vi "findAndTargetNeuronsNew.vi"() -> ()   [LabVIEW 2017]
uses:
  opencvSegmentConvertCoordinates-multiFrames.vi
  opencvSegmentConvertCoordinates-singleFrame.vi
  opencvSelectCandidateNeurons5Planes.vi
  opencvSegment.vi
  getComputerName.vi
  globalDevices.vi
  globalUtilities.vi
panel:
  in  "piezo1":dbl
  in  "piezo2":dbl
  in  "y":dbl
  in  "Numeric":i32=10 min=1
  in  "scale":dbl[](array[numeric])=[0.8, 0.5, 0.3]
  in  "lambda":dbl[](array[numeric])=[0.0, 0.0, 0.0]
  in  "stop 2":bool
  in  "stop":bool
  out "XY":u16[][][](array[numeric])
  out "XYZ":i32[][](array[numeric])
  out "curr. piezo pos (index)":i32
  in  "piezo M-1":i32=20
  in  "frames per second":dbl=20.0
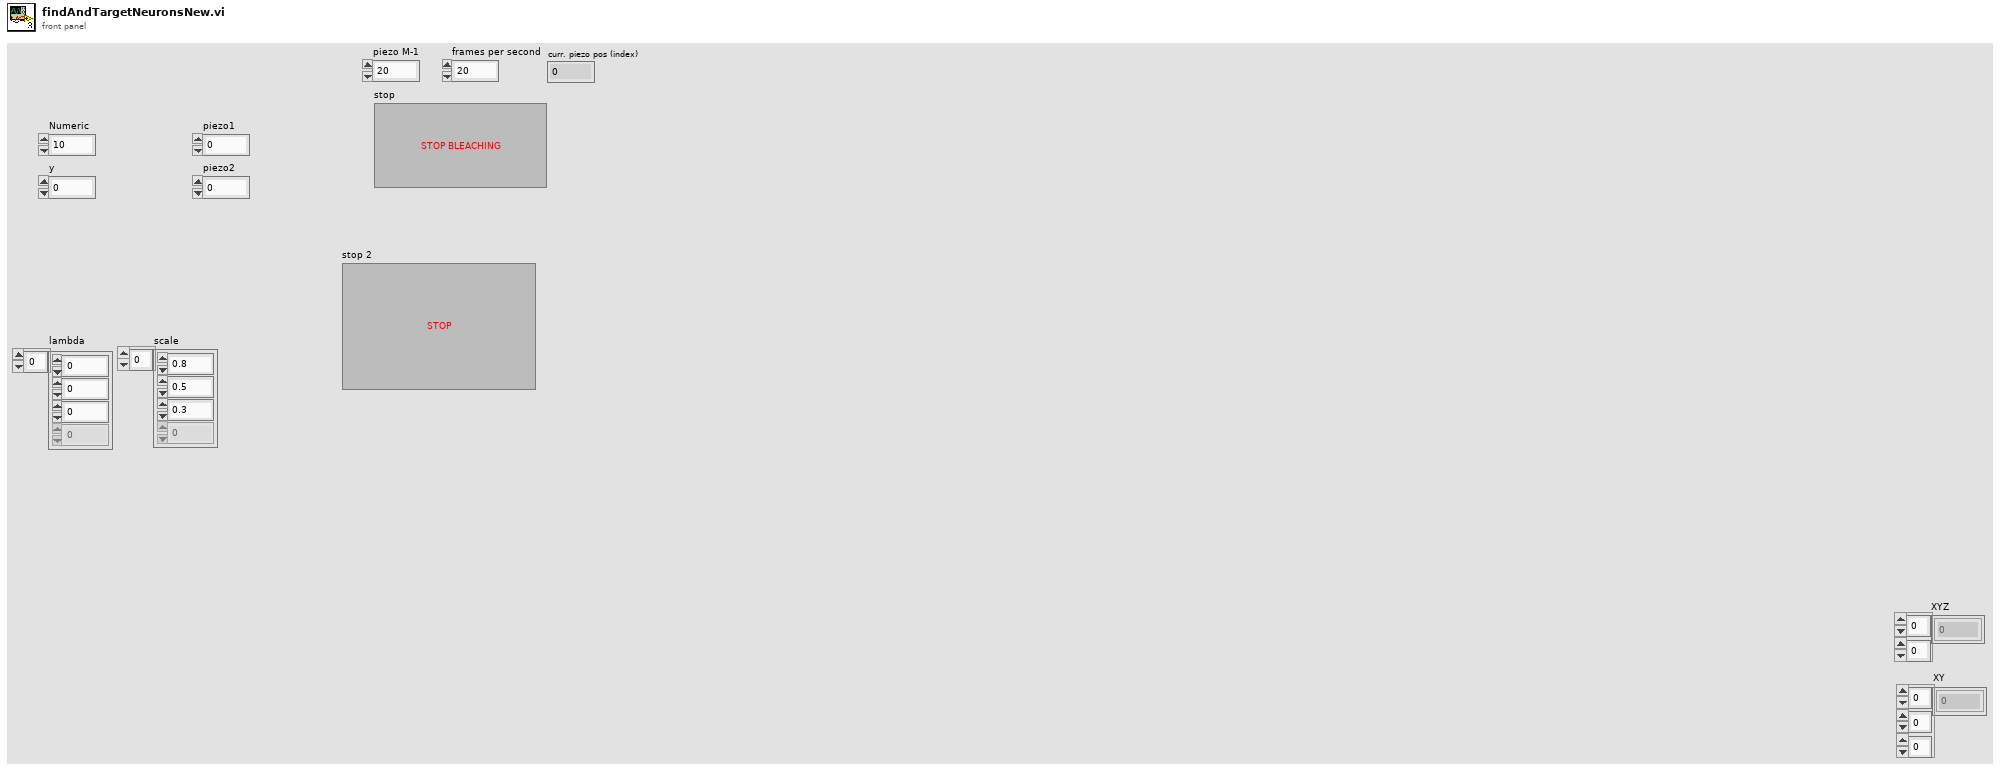
[diagram p1: front panel]
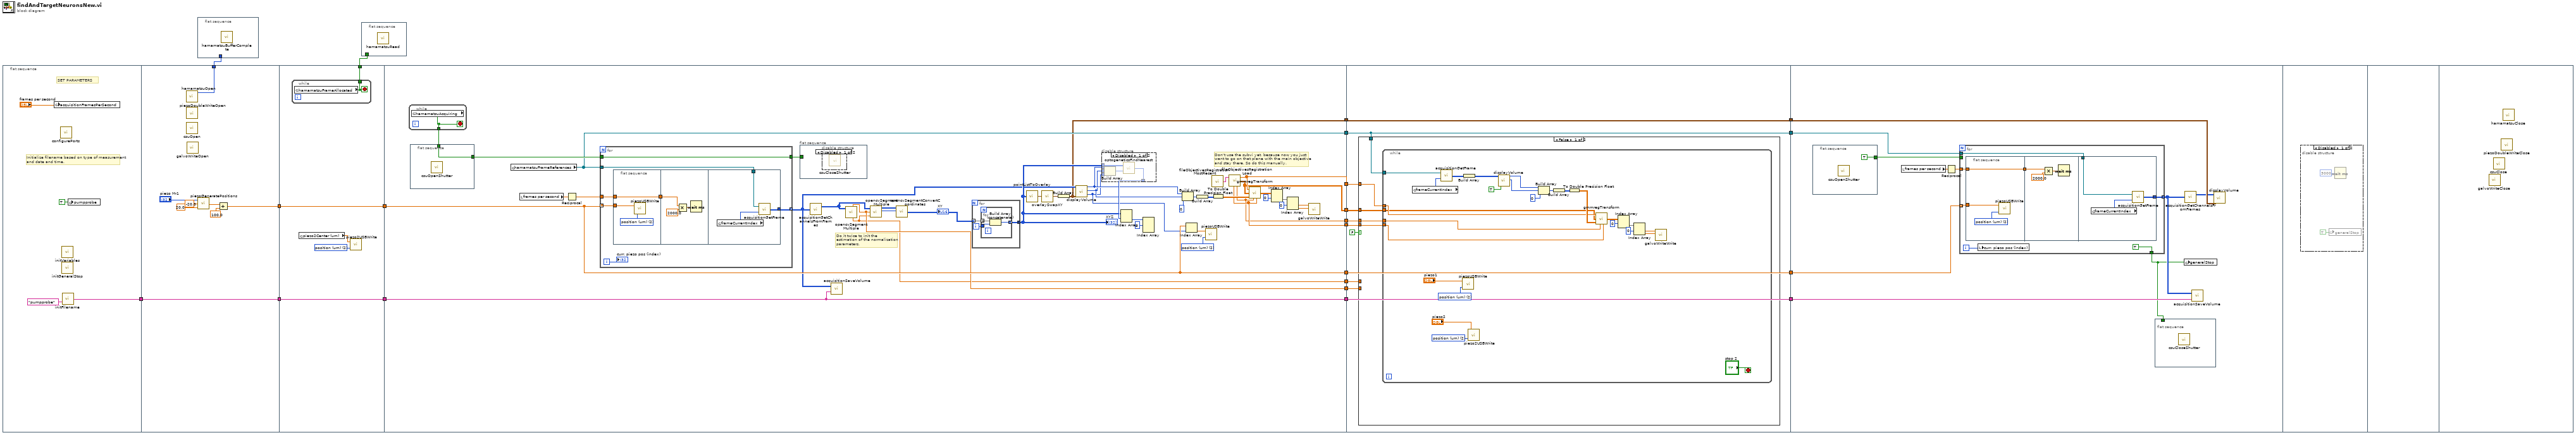
[diagram p0: block diagram]
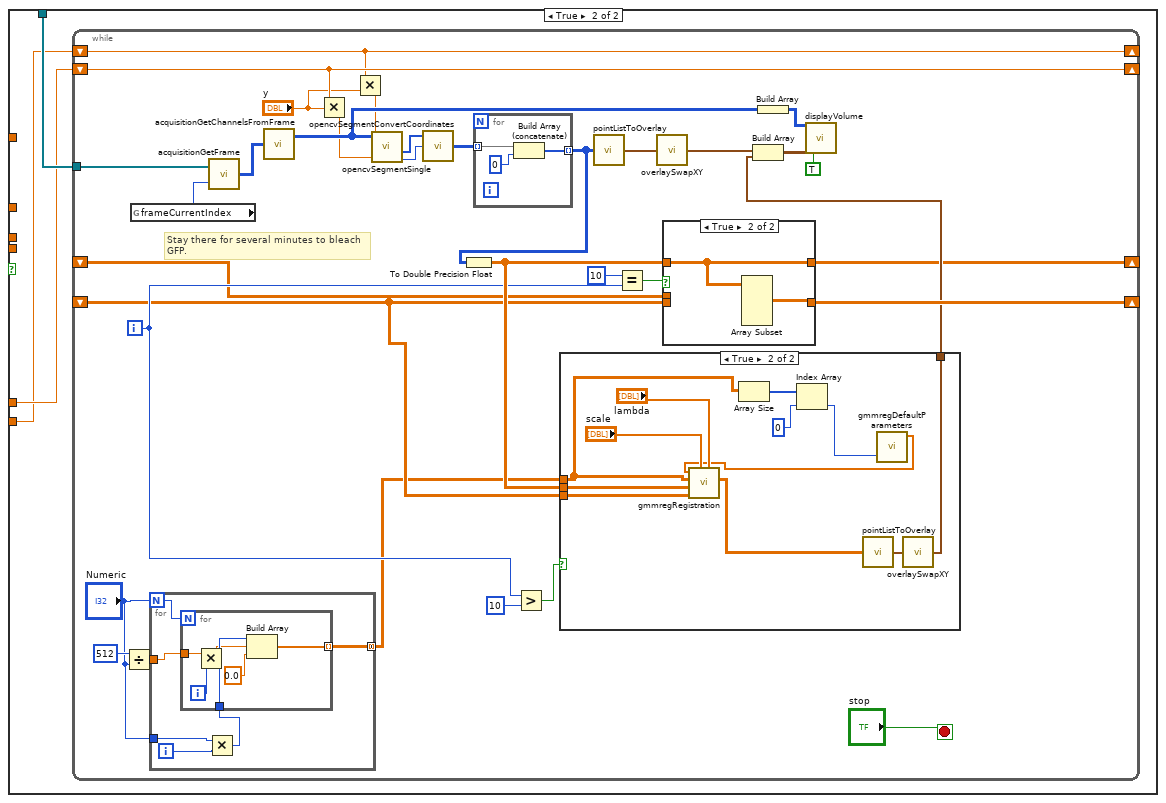
[diagram p4: hidden frame]
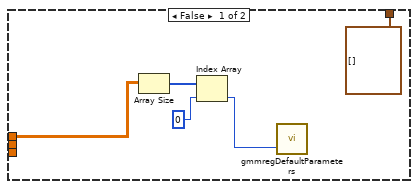
[diagram p5: hidden frame]
diagram:
  n1 = flat-sequence {
    tunnel: [w23] -> w16
    tunnel: [w28] -> w21
    tunnel: [w27] -> w19
    tunnel: [w26] -> w17
    tunnel: w16 -> [w26]
    tunnel: [w36] -> w20
    tunnel: w19 -> [w36]
    tunnel: [w35] -> w18
    tunnel: w17 -> [w35]
    tunnel: [w34] -> w7
    tunnel: w20 -> [w54]
    tunnel: w18 -> [w53]
    tunnel: [w55] -> w14
    tunnel: [w54] -> w12
    tunnel: [w53] -> w11
    tunnel: [w44] -> w9
    tunnel: [w46] -> w6
    tunnel: [w47] -> w5
    tunnel: [w43] -> w4
    tunnel: [w42] -> w3
    tunnel: [w41] -> w2
    tunnel: [w40] -> w1
    tunnel: [w120] -> w15
    tunnel: w14 -> [w120]
    tunnel: [w112] -> w13
    tunnel: w12 -> [w112]
    tunnel: w11 -> [w122]
    tunnel: [w122] -> w10
    tunnel: w9 -> [w121]
    tunnel: [w121] -> w8
    tunnel: w6 -> [w119]
    tunnel: w5 -> [w118]
    tunnel: w4 -> [w116]
    tunnel: w3 -> [w115]
    tunnel: w2 -> [w114]
    tunnel: w1 -> [w113]
    tunnel: w15 -> [w236]
    tunnel: w13 -> [w235]
    tunnel: w10 -> [w234]
    tunnel: w8 -> [w233]
    frame #0 {
      # "SET PARAMETERS"
      # "Initialize filename based on type of measurement\nand date and time."
      n2 = global write "globalUtilities.vi" "acquisitionFramesPerSecond"("frames per second") -> ()
      n3 = call "configurePorts.vi"() -> ()  [unwired: 12 in]
      n4 = call "initVariables.vi"() -> ()  [unwired: 12 in]
      n5 = call "initGeneralStop.vi"() -> ()  [unwired: 1 in]
      n6 = call "initFilename.vi"("Experiment type"="pumpprobe") -> ("folder name"=w23:string)  [unwired: 1 in]
      n7 = global write "globalUtilities.vi" "pumpprobe"(TRUE ("pumpprobe")) -> ()
    }
    frame #1 {
      n8 = call "hamamatsuOpen.vi"() -> ("Handle out"=w28:u32)  [unwired: 3 out]
      n9 = call "piezoDoubleWriteOpen.vi"() -> ()  [unwired: 2 in]
      n10 = call "csuOpen.vi"() -> ()  [unwired: 14 in, 2 out]
      n11 = call "galvoWriteOpen.vi"() -> ()  [unwired: 12 in]
      n12 = call "piezoGeneratePositions.vi"("zf"=20.0, "z0"=-20.0, "M"="piezo M-1") -> ("positions (z)"=w30:dbl[])
      n13 = Add(x=w30, y=100.0) -> (x+y=w27:dbl[])
    }
    frame #2 {
      w38 = u16 2 items=["fractional", "voltage (V)", "position (um)"] ("mode")
      n14 = while {
        tunnel: [w39] -> w34
        stop <- w39 stop-if-true
        n15 = global read "globalDevices.vi" "hamamatsuFrameAllocated"() -> (w39:bool)
      }
      n16 = global read "globalDevices.vi" "piezo2Center (um)"() -> (w37:dbl)
      n17 = call "piezo2USBWrite.vi"("mode"=w38, "position"=w37) -> ()  [unwired: 1 in]
    }
    frame #3 {
      w68 = u16 2 items=["fractional", "voltage (V)", "position (um)"] ("mode")
      # "Don't use the subvi yet, because now you just\nwant to go on that plane with the main objective\nand stay there. So do this manually."
      # "Do it twice to init the\nestimation of the normalization \nparameters."
      n18 = while {
        tunnel: [w111] -> w77
        stop <- w111 stop-if-true
        n19 = global read "globalUtilities.vi" "hamamatsuAcquiring"() -> (w111:bool)
      }
      n20 = flat-sequence {
        tunnel: w77 -> [w88]
        tunnel: [w88] -> w76
        frame #0 {
          n21 = call "csuOpenShutter.vi"() -> ()  [unwired: 16 in]
        }
      }
      n22 = global read "globalDevices.vi" "hamamatsuFrameReferences"() -> (w55:refnum<data-value>[])
      n23 = local read "frames per second"() -> (w81:dbl)
      n24 = Reciprocal(x=w81) -> (1/x=w80:dbl)
      n25 = for {
        tunnel: w55 -> [w100]
        tunnel: w54 -> [w101] mode=indexing
        tunnel: w80 -> [w99]
        tunnel: [w97] -> w48 mode=indexing
        tunnel: w76 -> [w95]
        tunnel: [w95] -> w75
        i -> [w96]
        n26 = flat-sequence {
          tunnel: w101 -> [w103]
          tunnel: w99 -> [w104]
          tunnel: [w104] -> w98
          tunnel: w98 -> [w105]
          tunnel: w100 -> [w109]
          tunnel: [w108] -> w97
          frame #0 {
            w102 = u16 2 items=["fractional", "voltage (V)", "position (um)"] ("mode")
            n27 = call "piezoUSBWrite.vi"("mode"=w102, "position"=w103) -> ()  [unwired: 1 in]
          }
          frame #1 {
            n28 = Multiply(x=w105, y=2000.0) -> (x*y=w107:dbl)
            n29 = Wait (ms)(milliseconds to wait=w107) -> ()  [unwired: 1 out]
          }
          frame #2 {
            n30 = global read "globalUtilities.vi" "frameCurrentIndex"() -> (w110:i32)
            n31 = call "acquisitionGetFrame.vi"("index"=w110, "hamamatsuFrameReferences"=w109) -> ("frameOut"=w108:u16[][])
          }
        }
        "curr. piezo pos (index)" <- w96
      }
      n32 = flat-sequence {
        tunnel: w75 -> [_]
        frame #0 {
          n33 = disable-structure shown="Disabled" {
            frame Disabled {
              n34 = call "csuCloseShutter.vi"() -> ()  [unwired: 16 in]
            }
            frame Enabled {
            }
          }
        }
      }
      n35 = call "acquisitionGetChannelsFromFrames.vi"("frameIn"=w48) -> ("Red"=w73:u16[][][])  [unwired: 1 out]
      n36 = call "acquisitionSaveVolume.vi"("folder"=w53, "volume"=w48) -> ()  [unwired: 1 in]
      n37 = call "opencvSegmentMultiple.vi"("ImgIn"=w73) -> ("maxY"=w46:dbl, "maxX"=w47:dbl)  [unwired: 2 in, 4 out]
      n38 = call "opencvSegmentMultiple.vi"("maxYInStack"=w46, "maxXInStack"=w47, "ImgIn"=w73) -> ("NeuronN[frame]"=w79:u16[], "NeuronXY[frame]"=w78:u16[][])  [unwired: 4 out]
      n39 = call-poly "opencvSegmentConvertCoordinates.vi"("NeuronN"=w79, "NeuronXY"=w78) -> ("XY"=w74:u16[][][])  [unwired: 1 in]
      "XY" <- w74
      n40 = for {
        tunnel: w74 -> [w91] mode=indexing
        tunnel: [w90] -> w71 mode=concatenating
        i -> [w89]
        n41 = for {
          tunnel: w91 -> [w94] mode=indexing
          tunnel: [w92] -> w90 mode=indexing
          tunnel: w89 -> [w93]
          n42 = Build Array (concatenate)(w94, w93) -> (w92:i32[])
        }
      }
      "XYZ" <- w71
      n43 = call "pointListToOverlay.vi"("points"=w71) -> ("overlay (XYZ)"=w49:cluster{"X":i32, "Y":i32, "Z":i32}[])
      n44 = call "overlaySwapXY.vi"("overlay in"=w49) -> ("overlay out"=w45:cluster{"X":i32, "Y":i32, "Z":i32}[])
      n45 = Build Array(w45) -> (w44:cluster{"X":i32, "Y":i32, "Z":i32}[][])
      n46 = call "displayVolume.vi"("frames"=w48, "overlay (z:-1 all planes)"=w44) -> ("X0out"=w52:i32, "Y0out"=w51:i32, "zout (plane index)"=w50:i32)  [unwired: 12 in, 3 out]
      n47 = disable-structure shown="Disabled" {
        disable-tunnel: w52 -> [w87 _]
        disable-tunnel: w51 -> [w86 _]
        disable-tunnel: w50 -> [w85 _]
        disable-tunnel: [w83 _] -> w72
        disable-tunnel: w71 -> [w82 _]
        frame Disabled {
          n48 = Build Array(w87, w86, w85) -> (w84:i32[])
          n49 = call "optogeneticsFindNearest.vi"("point"=w84, "points"=w82) -> ("min index(es)"=w83:i32)
        }
        frame Enabled {
        }
      }
      n50 = Index Array(array=w71, index (row)=w72) -> (element=w70:i32[])  [unwired: 1 in]
      n51 = Index Array(array=w70, index #1=0 ("index")) -> ()  [unwired: 2 in, 3 out]
      n52 = Build Array(w52, w51, 0 ("element")) -> (w64:i32[])
      n53 = Index Array(array=w54, index=w50) -> (element=w69:dbl)
      n54 = Build Array(w64) -> (w63:i32[][])
      n55 = call "piezoUSBWrite.vi"("mode"=w68, "position"=w69) -> ()  [unwired: 1 in]
      n56 = call "fileObjectivesRegistrationMostRecent.vi"() -> ("f"=w67:string)  [unwired: 1 in]
      n57 = To Double Precision Float(number=w63) -> (double precision float=w62:dbl[][])
      n58 = call "fileObjectivesRegistrationLoad.vi"("objectiveRegistrationFilePath"=w67) -> ("denormParam"=w41:dbl[], "param"=w43:dbl[], "imaging (model)"=w42:dbl[][], "normParam"=w40:dbl[])  [unwired: 3 in, 2 out]
      n59 = call "gmmregTransform.vi"("param0"=w43, "ctrlPts"=w42, "pts"=w62, "normParams"=w40, "denormParams"=w41) -> ("out"=w61:dbl[][])  [unwired: 4 in]
      n60 = Index Array(array=w61, index (row)=0) -> (element=w59:dbl[])  [unwired: 1 in]
      n61 = Index Array(array=w59, index #1=0 ("index")) -> (element #1=w57:dbl, element #2=w56:dbl)  [unwired: 1 in]
      n62 = call "galvoWriteWrite.vi"("X"=w57, "Y"=w56) -> ()  [unwired: 4 in]
    }
    frame #4 {
      n63 = case shown="False" FALSE {
        tunnel: w120 -> [w127 w156]
        tunnel: w119 -> [_ w155]
        tunnel: w118 -> [_ w154]
        tunnel: w116 -> [w126 _]
        tunnel: w115 -> [w125 _]
        tunnel: w114 -> [w124 _]
        tunnel: w113 -> [w123 _]
        frame False {
          n64 = while {
            tunnel: w127 -> [w151]
            tunnel: w126 -> [w138]
            tunnel: w125 -> [w137]
            tunnel: w124 -> [w135]
            tunnel: w123 -> [w136]
            stop <- "stop 2" stop-if-true
            w129 = u16 2 items=["fractional", "voltage (V)", "position (um)"] ("mode")
            w131 = u16 2 items=["fractional", "voltage (V)", "position (um)"] ("mode")
            n65 = global read "globalUtilities.vi" "frameCurrentIndex"() -> (w152:i32)
            n66 = call "acquisitionGetFrame.vi"("index"=w152, "hamamatsuFrameReferences"=w151) -> ("frameOut"=w150:u16[][])
            n67 = call "piezoUSBWrite.vi"("mode"=w131, "position"="piezo1") -> ()  [unwired: 1 in]
            n68 = Build Array(w150) -> (w149:u16[][][])
            n69 = call "piezo2USBWrite.vi"("mode"=w129, "position"="piezo2") -> ()  [unwired: 1 in]
            n70 = call "displayVolume.vi"("frames"=w149, "stop immediately"=TRUE) -> ("X0out"=w134:i32, "Y0out"=w133:i32)  [unwired: 12 in, 4 out]
            n71 = Build Array(w134, w133, 0 ("element")) -> (w140:i32[])
            n72 = Build Array(w140) -> (w141:i32[][])
            n73 = To Double Precision Float(number=w141) -> (double precision float=w142:dbl[][])
            n74 = call "gmmregTransform.vi"("param0"=w138, "ctrlPts"=w137, "pts"=w142, "normParams"=w136, "denormParams"=w135) -> ("out"=w143:dbl[][])  [unwired: 4 in]
            n75 = Index Array(array=w143, index (row)=0) -> (element=w145:dbl[])  [unwired: 1 in]
            n76 = Index Array(array=w145, index #1=0 ("index")) -> (element #1=w147:dbl, element #2=w148:dbl)  [unwired: 1 in]
            n77 = call "galvoWriteWrite.vi"("X"=w147, "Y"=w148) -> ()  [unwired: 4 in]
          }
        }
        frame True {
          n78 = while {
            tunnel: w156 -> [w188]
            shift-right: [w160] -> _
            shift-left: w154 -> [w160]
            shift-right: [w161] -> _
            shift-left: w155 -> [w161]
            shift-right: [w172] -> _
            shift-left: _ -> [w167]
            shift-right: [w177] -> _
            shift-left: _ -> [w166]
            i -> [w170]
            stop <- "stop" stop-if-true
            # "Stay there for several minutes to bleach\nGFP."
            n79 = Divide(x=512, y="Numeric") -> (x/y=w164:dbl)
            n80 = global read "globalUtilities.vi" "frameCurrentIndex"() -> (w189:i32)
            n81 = for {
              N: "Numeric" -> [w196]
              tunnel: w164 -> [w195]
              tunnel: "Numeric" -> [w193]
              tunnel: [w191] -> w162 mode=concatenating
              i -> [w194]
              n82 = Multiply(x=w193, y=w194) -> (x*y=w192:i32)
              n83 = for {
                N: w196 -> [_]
                tunnel: w192 -> [w200]
                tunnel: w195 -> [w198]
                tunnel: [w197] -> w191 mode=indexing
                i -> [w201]
                n84 = Multiply(x=w198, y=w201) -> (x*y=w199:dbl)
                n85 = Build Array(w200, w199, 0.0 ("element")) -> (w197:dbl[])
              }
            }
            n86 = call "acquisitionGetFrame.vi"("index"=w189, "hamamatsuFrameReferences"=w188) -> ("frameOut"=w187:u16[][])
            n87 = call "acquisitionGetChannelsFromFrame.vi"("frameIn"=w187) -> ("Red"=w184:u16[][])  [unwired: 1 out]
            n88 = Multiply(x=w161, y="y") -> (x*y=w158:dbl)
            n89 = Multiply(x=w160, y="y") -> (x*y=w159:dbl)
            n90 = call "opencvSegmentSingle.vi"("maxYInStack"=w158, "maxXInStack"=w159, "ImgIn"=w184) -> ("NeuronN[last frame]"=w181:u16, "NeuronXY[last frame]"=w182:u16[])  [unwired: 2 in, 2 out]
            n91 = call-poly "opencvSegmentConvertCoordinates.vi"("NeuronN"=w181, "NeuronXY"=w182) -> ("XY"=w180:u16[][])  [unwired: 1 in]
            n92 = for {
              tunnel: w180 -> [w226] mode=indexing
              tunnel: [w224] -> w173 mode=indexing
              n93 = Build Array (concatenate)(w226, 0) -> (w224:i32[])
            }
            n94 = To Double Precision Float(number=w173) -> (double precision float=w178:dbl[][])
            n95 = Greater?(x=w170, y=10) -> (0:w168:bool)
            n96 = case shown="True" w168 {
              tunnel: w178 -> [_ w218]
              tunnel: w162 -> [w203 w209]
              tunnel: w166 -> [_ w217]
              tunnel: [cluster{"X":i32, "Y":i32, "Z":i32}[] [] ("overlay out") w215] -> w175
              frame False {
                n97 = Array Size(array=w203) -> (size(s)=w206:i32[])
                n98 = Index Array(array=w206, index=0 ("index (row)")) -> (element=w204:i32)
                n99 = call "gmmregDefaultParameters.vi"("nctrlPts"=w204) -> ()  [unwired: 1 in, 4 out]
              }
              frame True {
                n100 = Array Size(array=w209) -> (size(s)=w212:i32[])
                n101 = Index Array(array=w212, index=0 ("index (row)")) -> (element=w210:i32)
                n102 = call "gmmregDefaultParameters.vi"("nctrlPts"=w210) -> ("param0"=w208:dbl[])  [unwired: 1 in, 3 out]
                n103 = call "gmmregRegistration.vi"("lambda"="lambda", "scale"="scale", "scene"=w217, "model"=w218, "ctrlPoints"=w209, "param0"=w208) -> ("out"=w214:dbl[][])  [unwired: 2 in, 3 out]
                n104 = call "pointListToOverlay.vi"("points"=w214) -> ("overlay (XYZ)"=w216:cluster{"X":i32, "Y":i32, "Z":i32}[])
                n105 = call "overlaySwapXY.vi"("overlay in"=w216) -> ("overlay out"=w215:cluster{"X":i32, "Y":i32, "Z":i32}[])
              }
            }
            n106 = call "pointListToOverlay.vi"("points"=w173) -> ("overlay (XYZ)"=w186:cluster{"X":i32, "Y":i32, "Z":i32}[])
            n107 = Equal?(x=10, y=w170) -> (x = y?=w179:bool)
            n108 = call "overlaySwapXY.vi"("overlay in"=w186) -> ("overlay out"=w176:cluster{"X":i32, "Y":i32, "Z":i32}[])
            n109 = case shown="True" w179 {
              tunnel: w178 -> [_ w223]
              tunnel: [w221 w223] -> w172
              tunnel: w167 -> [w221 _]
              tunnel: [w220 w222] -> w177
              tunnel: w166 -> [w220 _]
              frame False {
              }
              frame True {
                n110 = Array Subset(array=w223) -> (w222:dbl[][])  [unwired: 4 in]
              }
            }
            n111 = Build Array(w176, w175) -> (w174:cluster{"X":i32, "Y":i32, "Z":i32}[][])
            n112 = Build Array(w184) -> (w183:u16[][][])
            n113 = call "displayVolume.vi"("frames"=w183, "overlay (z:-1 all planes)"=w174, "stop immediately"=TRUE) -> ()  [unwired: 11 in, 6 out]
          }
        }
      }
    }
    frame #5 {
      n114 = flat-sequence {
        tunnel: [TRUE] -> w228
        frame #0 {
          n115 = call "csuOpenShutter.vi"() -> ()  [unwired: 16 in]
        }
      }
      n116 = local read "frames per second"() -> (w232:dbl)
      n117 = Reciprocal(x=w232) -> (1/x=w231:dbl)
      n118 = for {
        tunnel: w236 -> [w240]
        tunnel: w231 -> [w241]
        tunnel: w235 -> [w243] mode=indexing
        tunnel: [w239] -> w230 mode=indexing
        tunnel: [TRUE] -> w227
        tunnel: w228 -> [_]
        i -> [w238]
        n119 = flat-sequence {
          tunnel: w243 -> [w245]
          tunnel: [w244] -> w242
          tunnel: w241 -> [w244]
          tunnel: w242 -> [w249]
          tunnel: w240 -> [w251]
          tunnel: [w250] -> w239
          frame #0 {
            w246 = u16 2 items=["fractional", "voltage (V)", "position (um)"] ("mode")
            n120 = call "piezoUSBWrite.vi"("mode"=w246, "position"=w245) -> ()  [unwired: 1 in]
          }
          frame #1 {
            n121 = Multiply(x=w249, y=2000.0) -> (x*y=w247:dbl)
            n122 = Wait (ms)(milliseconds to wait=w247) -> ()  [unwired: 1 out]
          }
          frame #2 {
            n123 = global read "globalUtilities.vi" "frameCurrentIndex"() -> (w252:i32)
            n124 = call "acquisitionGetFrame.vi"("index"=w252, "hamamatsuFrameReferences"=w251) -> ("frameOut"=w250:u16[][])
          }
        }
        n125 = local write "curr. piezo pos (index)"(w238) -> ()
      }
      n126 = flat-sequence {
        tunnel: w227 -> [_]
        frame #0 {
          n127 = call "csuCloseShutter.vi"() -> ()  [unwired: 16 in]
        }
      }
      n128 = global write "globalUtilities.vi" "generalStop"(w227) -> ()
      n129 = call "acquisitionGetChannelsFromFrames.vi"("frameIn"=w230) -> ("Red"=w229:u16[][][])  [unwired: 1 out]
      n130 = call "acquisitionSaveVolume.vi"("folder"=w234, "volume"=w230) -> ()  [unwired: 1 in]
      n131 = call "displayVolume.vi"("frames"=w229, "overlay (z:-1 all planes)"=w233) -> ()  [unwired: 12 in, 6 out]
    }
    frame #6 {
      n132 = disable-structure shown="Disabled" {
        frame Disabled {
          n133 = global write "globalUtilities.vi" "generalStop"(TRUE ("generalStop")) -> ()
          n134 = Wait (ms)(milliseconds to wait=u32 3000) -> ()  [unwired: 1 out]
        }
        frame Enabled {
        }
      }
    }
    frame #7 {
    }
    frame #8 {
      n135 = call "galvoWriteClose.vi"() -> ()  [unwired: 12 in]
      n136 = call "csuClose.vi"() -> ()  [unwired: 12 in]
      n137 = call "piezoDoubleWriteClose.vi"() -> ()  [unwired: 1 in]
      n138 = call "hamamatsuClose.vi"() -> ()  [unwired: 1 out]
    }
  }
  n139 = flat-sequence {
    tunnel: w21 -> [_]
    frame #0 {
      n140 = call "hamamatsuBufferComplete.vi"() -> ()  [unwired: 12 in]
    }
  }
  n141 = flat-sequence {
    tunnel: w7 -> [_]
    frame #0 {
      n142 = call "hamamatsuRead.vi"() -> ()  [unwired: 12 in]
    }
  }
